vi "Teleop Intake Control.vi"(1 "Manipulator Button Cluster":T2, 2 "Manipulator Axes":T1, 3 "Driver Axes":T1) -> ()   [LabVIEW 2015]
uses:
  Common Code/Gamepads/Button Cluster.ctl
  Common Code/Gamepads/Axes Cluster.ctl
  Common Code/Intake Commands.ctl
  Common Code/Change Detect Boolean.vi
  Robot Global Data.vi
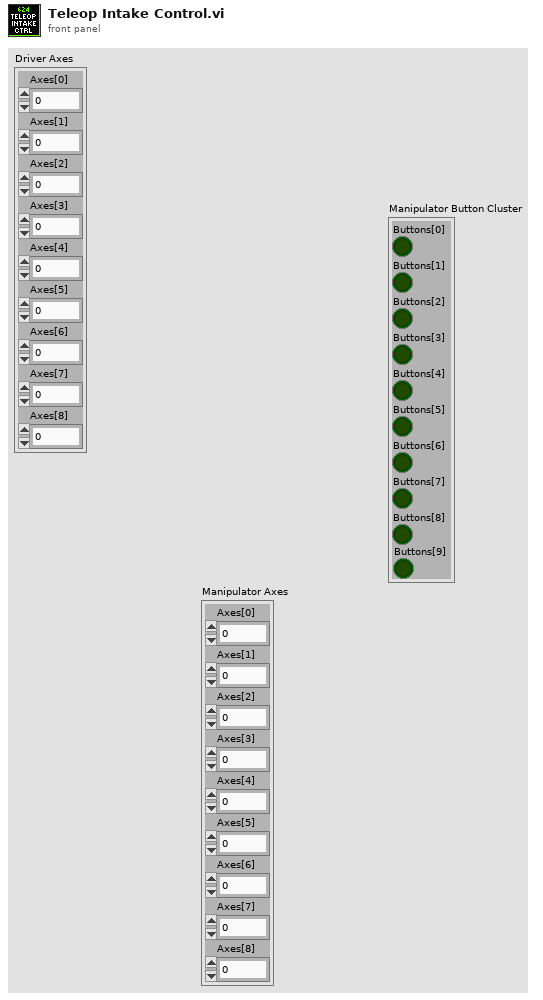
[diagram p1: front panel]
types:
  T1 = typedef "Axes Cluster.ctl" = cluster{"Axes[0]":dbl, "Axes[1]":dbl, "Axes[2]":dbl, "Axes[3]":dbl, "Axes[4]":dbl, "Axes[5]":dbl, "Axes[6]":dbl, "Axes[7]":dbl, "Axes[8]":dbl}
  T2 = typedef "Button Cluster.ctl" = cluster{"Buttons[0]":bool, "Buttons[1]":bool, "Buttons[2]":bool, "Buttons[3]":bool, "Buttons[4]":bool, "Buttons[5]":bool, "Buttons[6]":bool, "Buttons[7]":bool, "Buttons[8]":bool, "Buttons[9]":bool}
  T3 = typedef "Intake Commands.ctl" = enum16{"Settle Ball", "Unload", "Load", "Pull up", "Drop low", "Idle", "Lift Half", "Go To Angle"}
  T4 = enum16{"0", "1", "2", "3", "4", "5", "6", "7", "8", "9", "A", "B", "C", "D", "E", "F", "G", "H", "I", "J", "K", "L", "M", "N", "O", "P", "Q", "R", "S", "T", "U", "V", "W", "X", "Y", "Z", "F1", "F2", "F3", "F4", "F5", "F6", "F7", "F8", "F9", "F10", "F11", "F12", "F13", "F14", "F15", "ADD", "BACK", "BACKSLASH", "CAPITAL", "COMMA", "DECIMAL", "DELETE", "DIVIDE", "DOWN", "END", "EQUALS", "ESCAPE", "GRAVE (`)", "HOME", "INSERT", "LBRACKET", "LCONTROL", "LEFT", "L ALT", "LSHIFT", "LWIN", "MINUS", "MULTIPLY", "NEXT", "NUMLOCK", "NUMPAD_0", "NUMPAD_1", "NUMPAD_2", "NUMPAD_3", "NUMPAD_4", "NUMPAD_5", "NUMPAD_6", "NUMPAD_7", "NUMPAD_8", "NUMPAD_9", "PAUSE", "PERIOD", "PRIOR (PG UP)", "RBRACKET", "RCONTROL", "RETURN", "RIGHT", "R ALT", "RSHIFT", "RWIN", "SCROLL", "SEMICOLON", "SLASH", "SPACE", "SUBTRACT", "TAB", "UP", "ENTER (num pad)", "' (quote)"}
  T5 = typedef "Intake Mode.ctl" = enum16{"Safe", "Auto", "Manual"}
  T6 = typedef "Intake Commands Cluster.ctl" = cluster{"Intake Commands":T3, "Intake Mode":T5, "Override IR":bool, "Angle Target":dbl}
  T7 = typedef "Manual Intake Commands.ctl" = cluster{"Intake":bool, "Eject":bool, "Arm Angle":dbl, "Intake Override Speed":dbl, "Arm Override Speed":dbl, "Arm Speed":dbl, "Override Intake":bool, "Override Eject":bool, "Eject Override Speed":dbl, "Arm":bool, "Override Arm":bool, "Override Angle":bool}
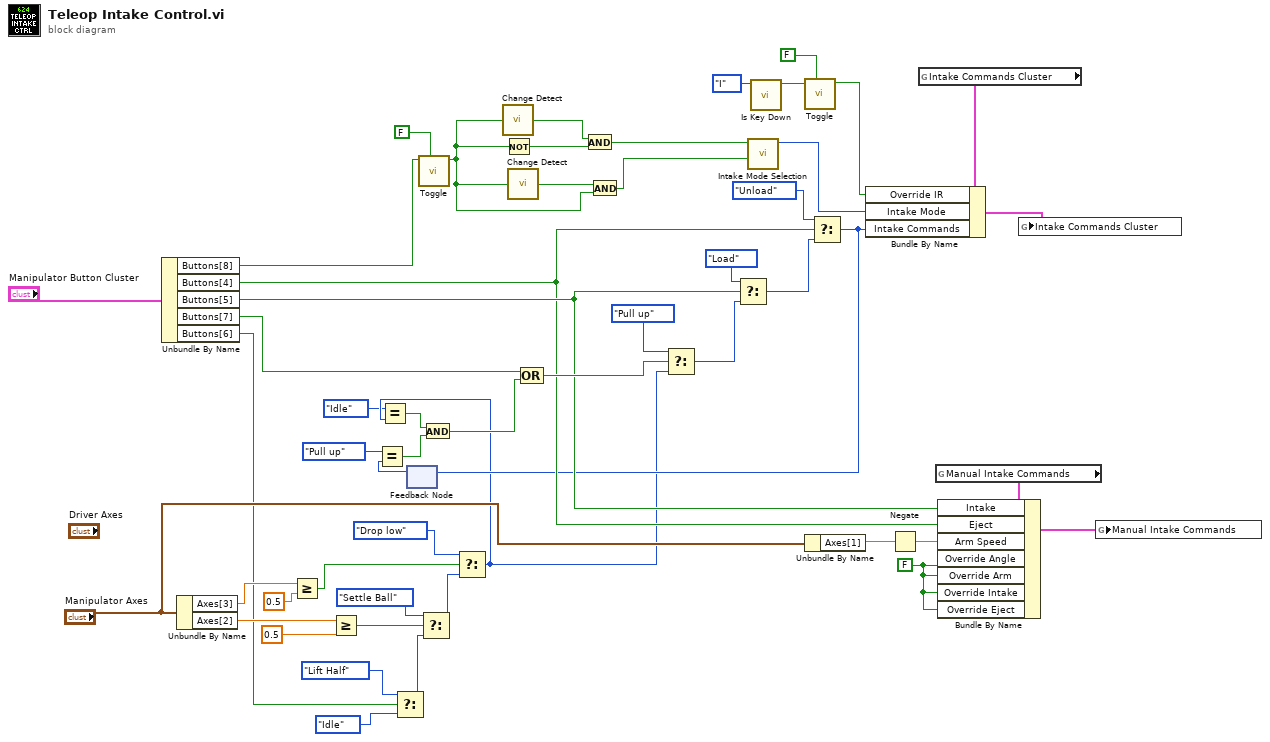
[diagram p0: block diagram]
diagram:
  w22 = FALSE ("Override Angle")
  n1 = Unbundle By Name("Manipulator Button Cluster") -> ("Buttons[8]"=w8:bool, "Buttons[4]"=w32:bool, "Buttons[5]"=w34:bool, "Buttons[7]"=w31:bool, "Buttons[6]"=w13:bool)
  n2 = Unbundle By Name("Manipulator Axes") -> ("Axes[3]"=w46:dbl, "Axes[2]"=w42:dbl)
  n3 = Greater Or Equal?(x=w46, y=0.5) -> (x >= y?=w33:bool)
  n4 = Greater Or Equal?(x=w42, y=0.5) -> (x >= y?=w11:bool)
  n5 = Select(t=Intake_Commands."Lift Half" ("f"), s=w13, f=Intake_Commands."Idle") -> (s? t:f=w12:T3)
  n6 = feedback #1() -> (w21:T3)  [unwired: 1 in]
  n7 = Equal?(x=Intake_Commands."Pull up", y=w21) -> (x = y?=w18:bool)
  n8 = call "Toggle.vi"("Initial Value"=FALSE, "In"=w8) -> ("Toggled"=w1:bool)  [unwired: 9 in]
  n9 = Select(t=Intake_Commands."Settle Ball", s=w11, f=w12) -> (s? t:f=w9:T3)
  n10 = Select(t=Intake_Commands."Drop low" ("Intake Commands"), s=w33, f=w9) -> (s? t:f=w15:T3)
  n11 = Equal?(x=Intake_Commands."Idle", y=w15) -> (x = y?=w19:bool)
  n12 = And(x=w19, y=w18) -> (x .and. y?=w17:bool)
  n13 = call-poly "Change Detect.vi"("In"=w1) -> ("Changed?"=w7:bool)
  n14 = Not(x=w1) -> (.not. x?=w5:bool)
  n15 = call-poly "Change Detect.vi"("In"=w1) -> ("Changed?"=w3:bool)
  n16 = Compound Arithmetic op=OR(w31, w17) -> (w38:bool)
  n17 = And(x=w7, y=w5) -> (x .and. y?=w4:bool)
  n18 = And(x=w3, y=w1) -> (x .and. y?=w2:bool)
  n19 = Select(t=Intake_Commands."Pull up" ("Intake Commands"), s=w38, f=w15) -> (s? t:f=w49:T3)
  n20 = Select(t=Intake_Commands."Load" ("Intake Commands"), s=w34, f=w49) -> (s? t:f=w40:T3)
  n21 = call "Intake Mode Selection.vi"("Set To Manual?"=w2, "Set To Auto?"=w4) -> ("Mode"=w35:T5)  [unwired: 9 in]
  n22 = call "Is Key Down.vi"("Key"=T4."I") -> ("Key Down?"=w30:bool)  [unwired: 10 in]
  n23 = call "Toggle.vi"("Initial Value"=FALSE, "In"=w30) -> ("Toggled"=w24:bool)  [unwired: 9 in]
  n24 = Unbundle By Name("Manipulator Axes") -> ("Axes[1]"=w36:dbl)
  n25 = Select(t=Intake_Commands."Unload" ("Intake Commands"), s=w32, f=w40) -> (s? t:f=w20:T3)
  n26 = feedback-in #1(w20) -> ()
  n27 = Negate(x=w36) -> (-x=w27:dbl)
  n28 = global read "Robot Global Data.vi" "Intake Commands Cluster"() -> (w48:T6)
  n29 = Bundle By Name(cluster=w48, "Override IR"=w24, "Intake Mode"=w35, "Intake Commands"=w20) -> (w47:T6)
  n30 = global read "Robot Global Data.vi" "Manual Intake Commands"() -> (w26:T7)
  n31 = Bundle By Name(cluster=w26, "Intake"=w34, "Eject"=w32, "Arm Speed"=w27, "Override Angle"=w22, "Override Arm"=w22, "Override Intake"=w22, "Override Eject"=w22) -> (w28:T7)
  n32 = global write "Robot Global Data.vi" "Intake Commands Cluster"(w47) -> ()
  n33 = global write "Robot Global Data.vi" "Manual Intake Commands"(w28) -> ()
